vi "Get__slk_mt.vi"(8 "error in (no error)":errorcluster, 11 "boolean in":refnum<class "Boolean__slk_mt.lvclass">) -> (0 "error out":errorcluster, 3 "boolean out":refnum<class "Boolean__slk_mt.lvclass">, 5 "value":string[](array[string]))   [LabVIEW 2011, in "Lazyboots Menu Tool.lvlib" / "Boolean__slk_mt.lvclass"]
doc: "Gets the value from the control on GUI.\n\n<b>Value:</b>\n[Section, Key, Value]"
uses:
  Boolean__slk_mt.lvclass
  Boolean__slk_mt.lvclass/Boolean__slk_mt.ctl
panel:
  # "Get__slk_mt.vi\nGets the values from the control on GUI.\n\nNOTICE -- YOU MUST LEAVE THIS NOTICE IN PLACE.\n\nCopyright (c) 2011, LIANG LIU Shawn.Liu.cn@gmail.com\nAll rights reserved.\n\nRedistribution and use in source and binary forms, with or without modification, are permitted provided that the following conditions are met:\n-Redistributions of source code must retain the above copyright notice, this list of conditions and the following disclaimer.\n-Redistributions in binary form must reproduce the above copyright notice, this list of conditions and the following disclaimer in the documentation and/or other materials provided with the distribution.\n-Neither the name of the eLp nor the names of its contributors may be used to endorse or promote products derived from this software without specific prior written permission.\n\nTHIS SOFTWARE IS PROVIDED BY THE COPYRIGHT HOLDERS AND CONTRIBUTORS \"AS IS\" AND ANY EXPRESS OR IMPLIED WARRANTIES, INCLUDING, BUT NOT LIMITED TO, THE IMPLIED WARRANTIES OF MERCHANTABILITY AND FITNESS FOR A PARTICULAR PURPOSE ARE DISCLAIMED. IN NO EVENT SHALL THE COPYRIGHT HOLDER OR CONTRIBUTORS BE LIABLE FOR ANY DIRECT, INDIRECT, INCIDENTAL, SPECIAL, EXEMPLARY, OR CONSEQUENTIAL DAMAGES (INCLUDING, BUT NOT LIMITED TO, PROCUREMENT OF SUBSTITUTE GOODS OR SERVICES; LOSS OF USE, DATA, OR PROFITS; OR BUSINESS INTERRUPTION) HOWEVER CAUSED AND ON ANY THEORY OF LIABILITY, WHETHER IN CONTRACT, STRICT LIABILITY, OR TORT (INCLUDING NEGLIGENCE OR OTHERWISE) ARISING IN ANY WAY OUT OF THE USE OF THIS SOFTWARE, EVEN IF ADVISED OF THE POSSIBILITY OF SUCH DAMAGE."
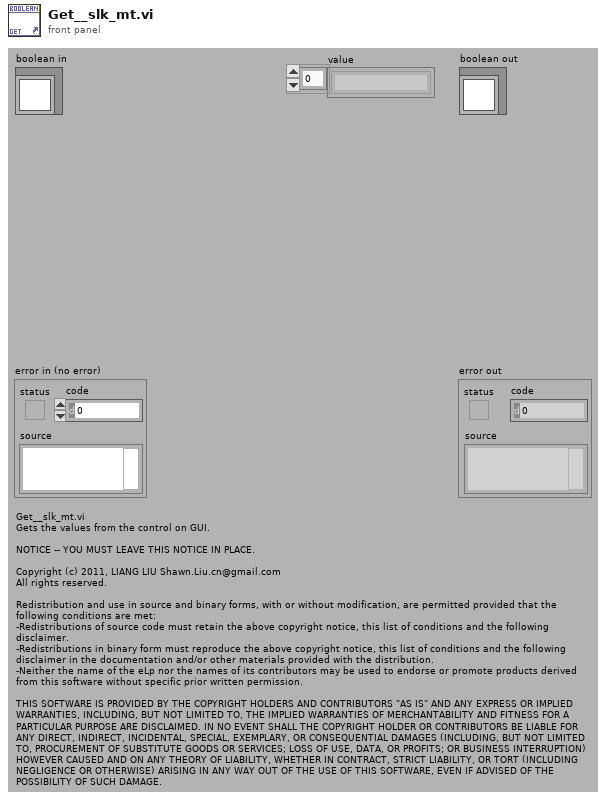
[diagram p1: front panel]
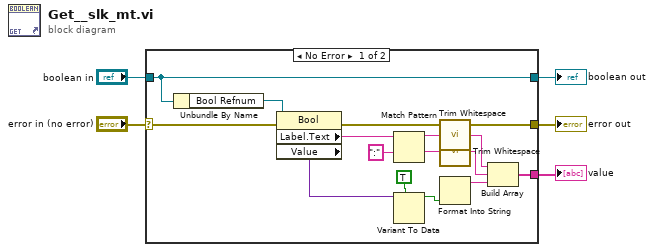
[diagram p0: block diagram]
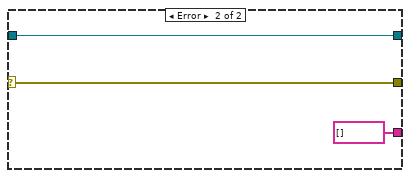
[diagram p2: hidden frame]
diagram:
  n1 = case shown="No Error" "error in (no error)" {
    selector: "error in (no error)" -> [w7 w23]
    tunnel: [w10 string[] []] -> w5
    tunnel: [w9 w23] -> w4
    tunnel: "boolean in" -> [w6 w22]
    tunnel: [w6 w22] -> w1
    frame No Error {
      n2 = Unbundle By Name(w6) -> ("Bool Refnum"=w8:refnum<vi>)
      n3 = property class="Bool"(reference=w8, error in=w7) -> (error out=w9:errorcluster, "Label.Text"=w20:string, "Value"=w16:variant)  [unwired: 1 out]
      n4 = Match Pattern(string=w20, regular expression=":") -> (before substring=w18:string, after substring=w17:string)  [unwired: 1 in, 2 out]
      n5 = Variant To Data(type=TRUE, Variant=w16) -> (data=w12:bool)  [unwired: 1 in, 1 out]
      n6 = call <vilib>:"Trim Whitespace.vi"("string"=w18) -> ("trimmed string"=w14:string)  [unwired: 1 in]
      n7 = call <vilib>:"Trim Whitespace.vi"("string"=w17) -> ("trimmed string"=w13:string)  [unwired: 1 in]
      n8 = Format Into String(w12) -> (resulting string=w11:string)  [unwired: 3 in, 1 out]
      n9 = Build Array(w14, w13, w11) -> (w10:string[])
    }
    frame Error {
    }
  }
  "error out" <- w4
  "boolean out" <- w1
  "value" <- w5
